vi "tt20_update_histogram_plot.vi"(8 "error in (no error)":errorcluster, 9 "histogram":cluster{dbl[], dbl[]}[](array[cluster]), 10 "tt20panel in":refnum<class "tt20panel.lvclass">, 11 "tt20 in":refnum<class "tt20.lvclass">) -> (0 "error out":errorcluster, 2 "panel out":refnum<class "tt20panel.lvclass">, 3 "tt20 out":refnum<class "tt20.lvclass">)   [LabVIEW 2015, in "tt20.lvclass"]
uses:
  tt20.lvclass
  tt20panel_class/tt20panel.lvclass
  UI/panel_class/panel.lvclass/panel.ctl
  UI/panel_class/panel.lvclass
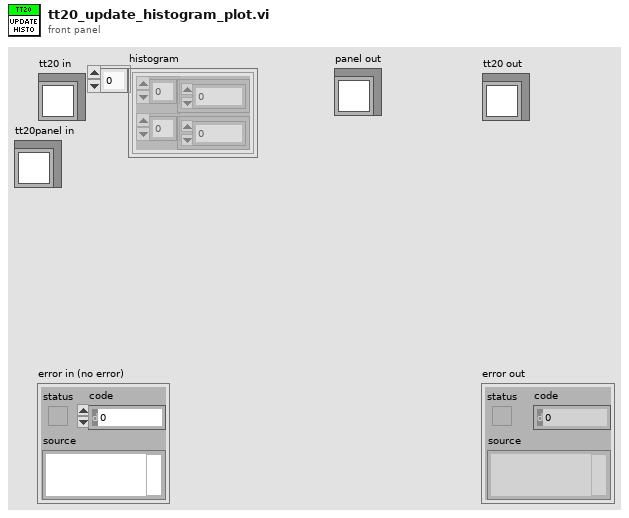
[diagram p1: front panel]
types:
  T1 = typedef "ui_user_events.ctl" = cluster{"update_xy_graph":refnum<user-event>, "update_graph":refnum<user-event>, "update_chart":refnum<user-event>, "update_map":refnum<user-event>, "event_loop_stop":refnum<user-event>, "keep_map":refnum<user-event>}
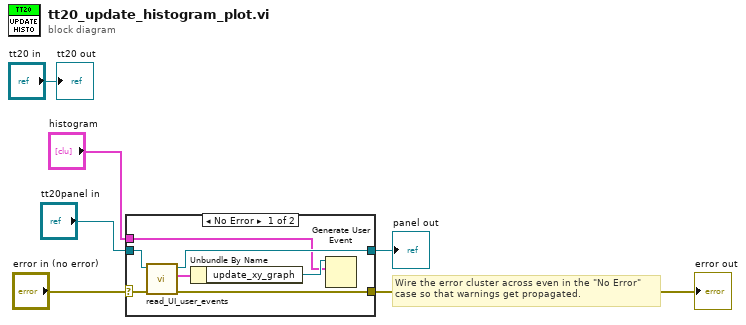
[diagram p0: block diagram]
diagram:
  # "Wire the error cluster across even in the \"No Error\"\ncase so that warnings get propagated."
  n1 = case shown="No Error" "error in (no error)" {
    selector: "error in (no error)" -> [w13 w15]
    tunnel: [w9 w15] -> w2
    tunnel: [w10 w14] -> w1
    tunnel: "tt20panel in" -> [w8 w14]
    tunnel: "histogram" -> [w7 _]
    frame No Error {
      n2 = call "read_UI_user_events.vi"("error in (no error)"=w13, "panel in"=w8) -> ("error out"=w9:errorcluster, "ui_user_events"=w12:T1, "panel out"=w10:refnum<class "tt20panel.lvclass">)  [unwired: 7 in]
      n3 = Unbundle By Name(w12) -> ("update_xy_graph"=w11:refnum<user-event>)
      n4 = Generate User Event(user event=w11, event data cluster=w7) -> ()  [unwired: 2 in, 2 out]
    }
    frame Error {
    }
  }
  "error out" <- w2
  "panel out" <- w1
  "tt20 out" <- "tt20 in"
